vi "Channel Performance Test.vi"() -> ()   [LabVIEW 2021]
uses:
  CIFUtilities/CIFChannels/Typedef/Channel State.ctl
  <vilib>/Platform/TimedLoop/XDataNode/timing_clust.ctl
  <vilib>/Platform/TimedLoop/XDataNode/nitl_modes.ctl
  <vilib>/Platform/TimedLoop/XDataNode/wakeup.ctl
  Double/RTFIFODouble.lvclass/RTFIFODouble.ctl
  CIFUtilities/CIFChannels/CIFChannels.lvclass/CIFChannels.ctl
  ecd22e40-9ef3-47c9-84dd-6e51471c5b7d.vi
  cc845de9-9662-4d69-8494-93190ebbf16f.vi
  5dde9a10-7574-45f3-be33-437a2b751792.vi
  630e717b-411c-4f0a-96f3-098c02e0b307.vi
  27ef35cb-55c2-4e73-bad1-dda663d636b9.vi
  <vilib>/Utility/error.llb/Clear Errors.vi
  CIFUtilities/CIFChannels/Accessors/Write Channel State.vi
  CIFUtilities/CIFChannels/Accessors/Read Direction.vi
  ecd22e40-9ef3-47c9-84dd-6e51471c5b7d.vi/c28b0ead-42ad-4072-80a2-aca7f2bd7ce3.vi
  cc845de9-9662-4d69-8494-93190ebbf16f.vi/4bc1c15b-36ab-481f-b8dd-c64075ce723a.vi
  cc845de9-9662-4d69-8494-93190ebbf16f.vi/d83cb72b-7713-41fc-a3d1-682de79cf574.vi
  5dde9a10-7574-45f3-be33-437a2b751792.vi/c28b0ead-42ad-4072-80a2-aca7f2bd7ce3.vi
  630e717b-411c-4f0a-96f3-098c02e0b307.vi/c28b0ead-42ad-4072-80a2-aca7f2bd7ce3.vi
  630e717b-411c-4f0a-96f3-098c02e0b307.vi/219d0231-d98b-4193-b5cc-84f90e3c9091.vi
  27ef35cb-55c2-4e73-bad1-dda663d636b9.vi/c28b0ead-42ad-4072-80a2-aca7f2bd7ce3.vi
  27ef35cb-55c2-4e73-bad1-dda663d636b9.vi/219d0231-d98b-4193-b5cc-84f90e3c9091.vi
  Double/RTFIFODouble.lvclass
  D:/dev/CIF-LVCore/src/CIFUtilities/CIFChannels/CIFChannels.lvclass
  CIF-Core-LabVIEW/src/CIFServices/CIFServices Fill In Error Info Ex.vi
  <vilib>/Platform/TimedLoop/XDataNode/XDataNode.xnode
  <vilib>/Platform/TimedLoop/XDataNode/XDNodeRunTimeDep.lvlib
  CIF-Core-LabVIEW/src/CIFServices/CifChannelServices.lvlib
  CIFUtilities/CIFChannels/CIFChannels.lvclass
panel:
  out "avg RTFIFO 2":dbl
  out "Max RTFIFO 2":dbl
  out "Numeric 6":i32
  out "Numeric 5":dbl
  out "Numeric 4":dbl
  out "Channel State":T1
  out "Numeric 3":dbl
  out "Numeric 2":dbl
  out "Numeric":i32
  out "avg channel":dbl
  out "max channel":dbl
  out "avg RTFIFO":dbl
  out "Max RTFIFO":dbl
  out "pass":bool
  out "error out":errorcluster
  # "This test should be run on RT.  It stresses the communications by constantly creating resource contraints with the low priority sender and the high priority loop. On Windows the priority of the loops cannot be set."
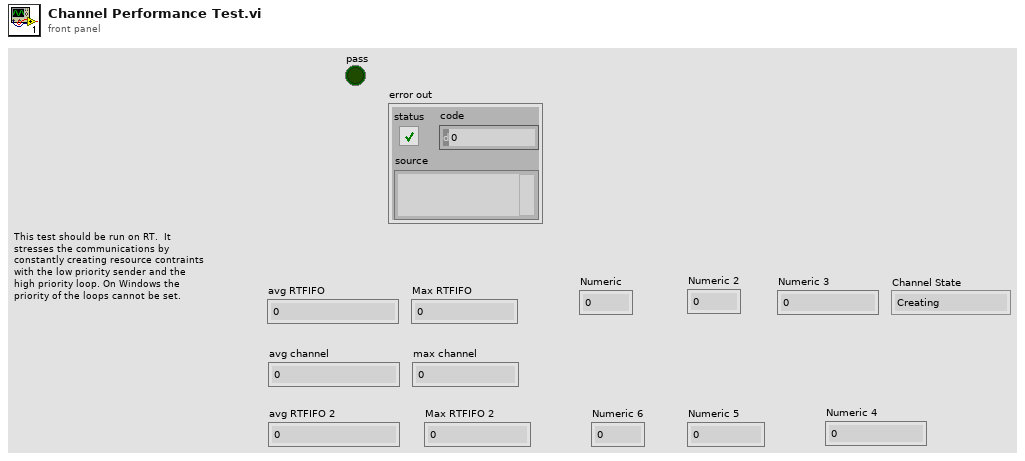
[diagram p1: front panel]
types:
  T1 = typedef "CIFChannels.lvclass/Channel State.ctl" = enum16{"Creating", "Disconnected", "Connecting", "Connected", "Destroying"}
  T2 = typedef "XDNodeRunTimeDep.lvlib/timing_clust.ctl" = cluster{"Expected End [f-1]":u64, "Actual End [f-1]":u64, "Finished Late? [f-1]":bool, "Expected End [i-1]":u64, "Actual End [i-1]":u64, "Finished Late? [i-1]":bool, "Expected Start [i]":u64, "Actual Start [i]":u64, "Expected Start [f]":u64, "Actual Start [f]":u64, "Source Name":string, "Structure Name":string, "Period":i64, "Deadline":i64, "Offset":i64, "Start":i64, "Priority":i32, "Timeout":i32, "Mode":T3, "Wakeup Reason":T4, "Error":errorcluster, "Source Type":string, "Secondary Source Type":string, "Global End Time":u64, "Global Start Time":u64, "Frame Duration":u64, "Iteration Duration":u64, "Assigned CPU":i32, "I/O Scan Engine Mode":u32}
  T3 = typedef "XDNodeRunTimeDep.lvlib/nitl_modes.ctl" = enum32{"No Change", "Process missed periods, maintain original phase", "Discard missed periods, maintain original phase", "Process missed periods, ignore original phase", "Discard missed periods, ignore original phase"}
  T4 = typedef "XDNodeRunTimeDep.lvlib/wakeup.ctl" = enum32{"Normal", "Aborted", "Asynchronous wakeup", "Timing source error", "Timed loop error", "Timeout"}
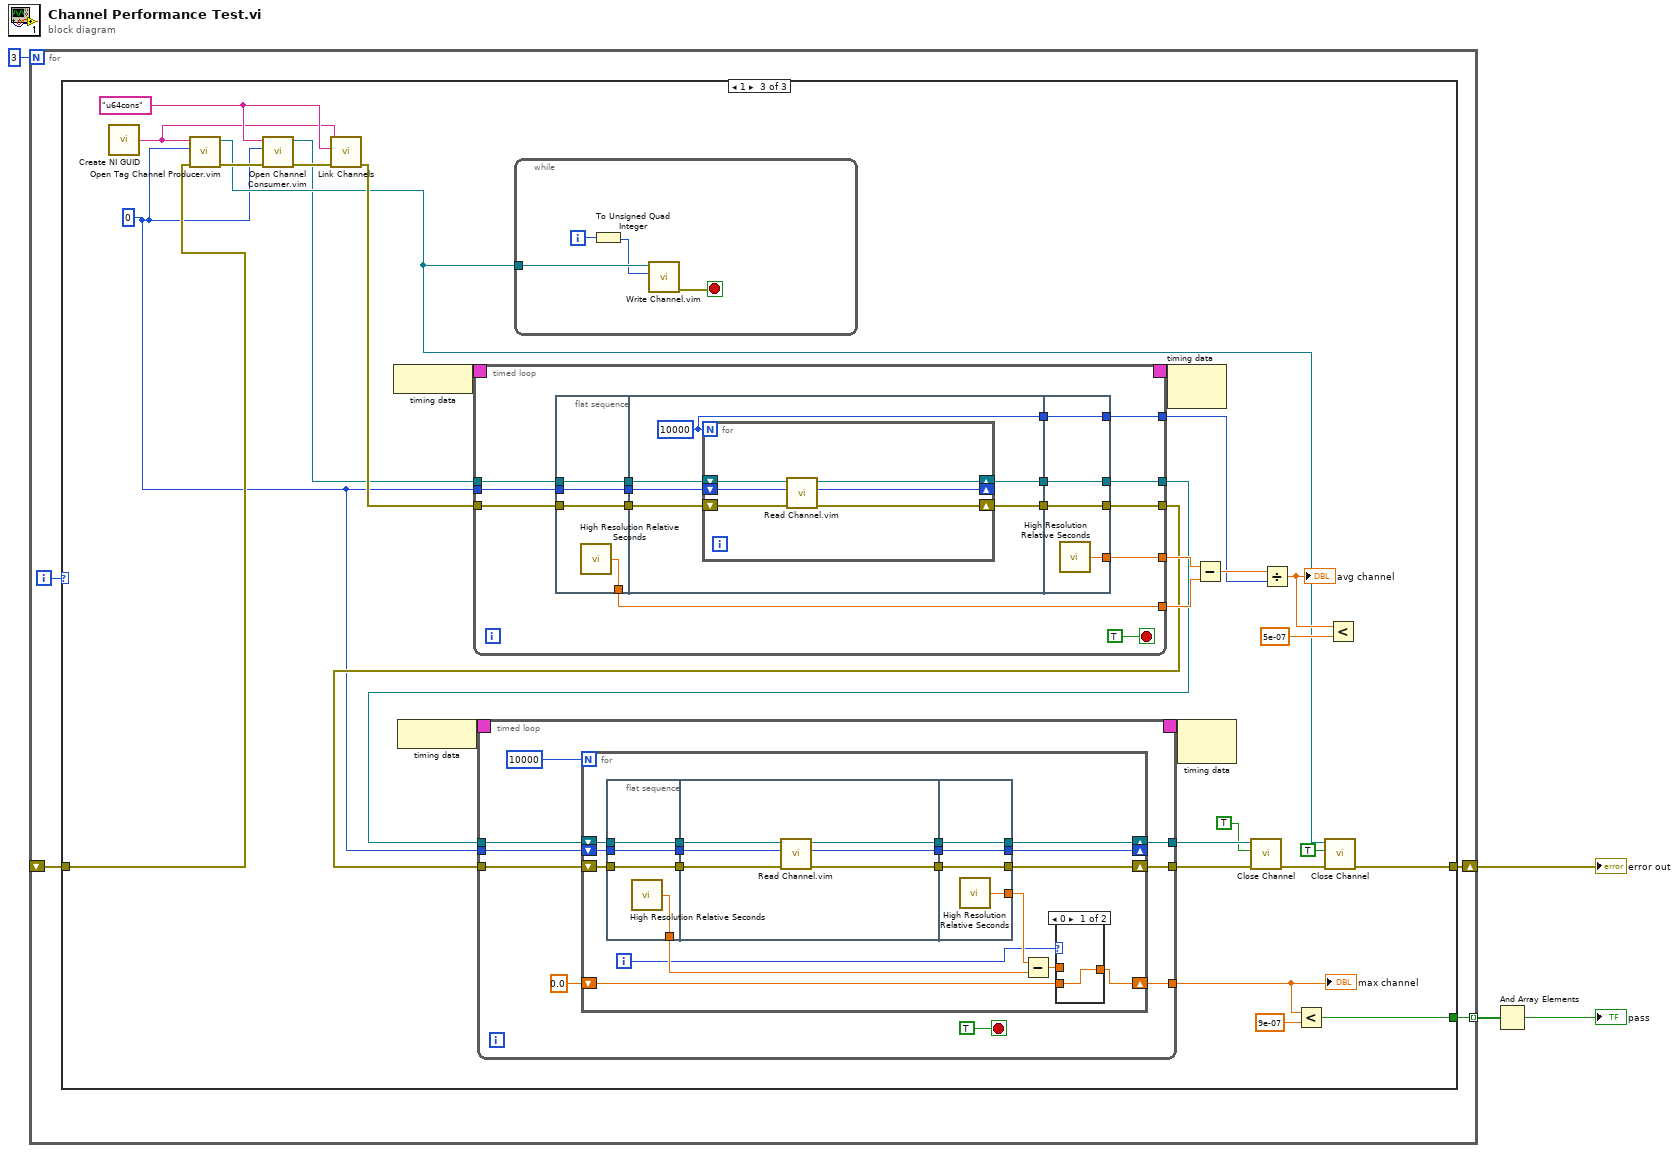
[diagram p0: block diagram]
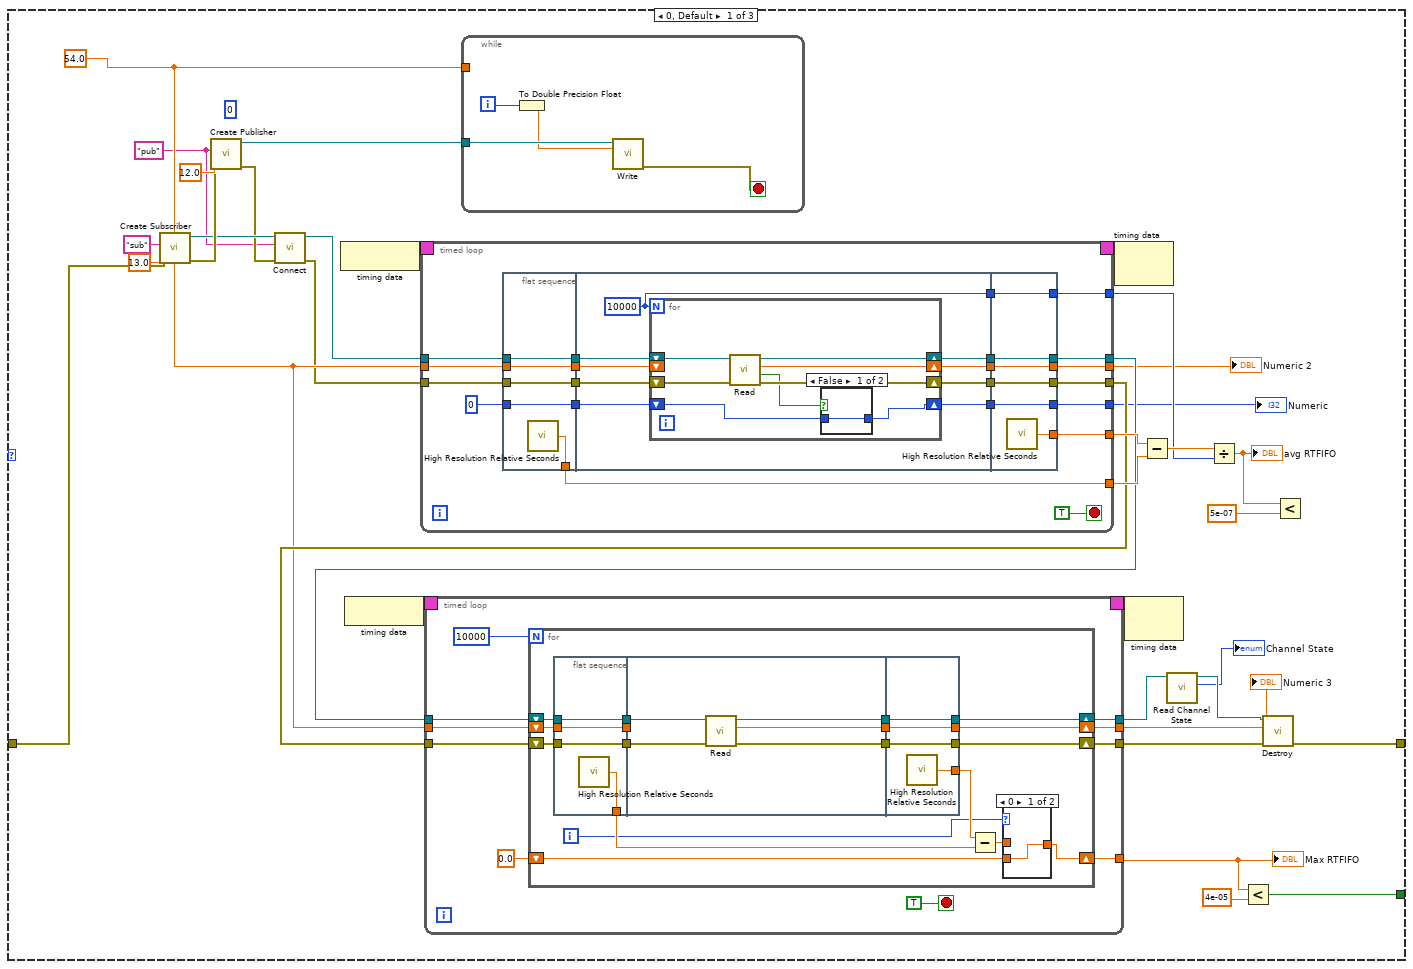
[diagram p2: hidden frame]
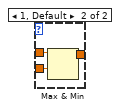
[diagram p3: hidden frame]
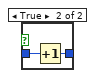
[diagram p4: hidden frame]
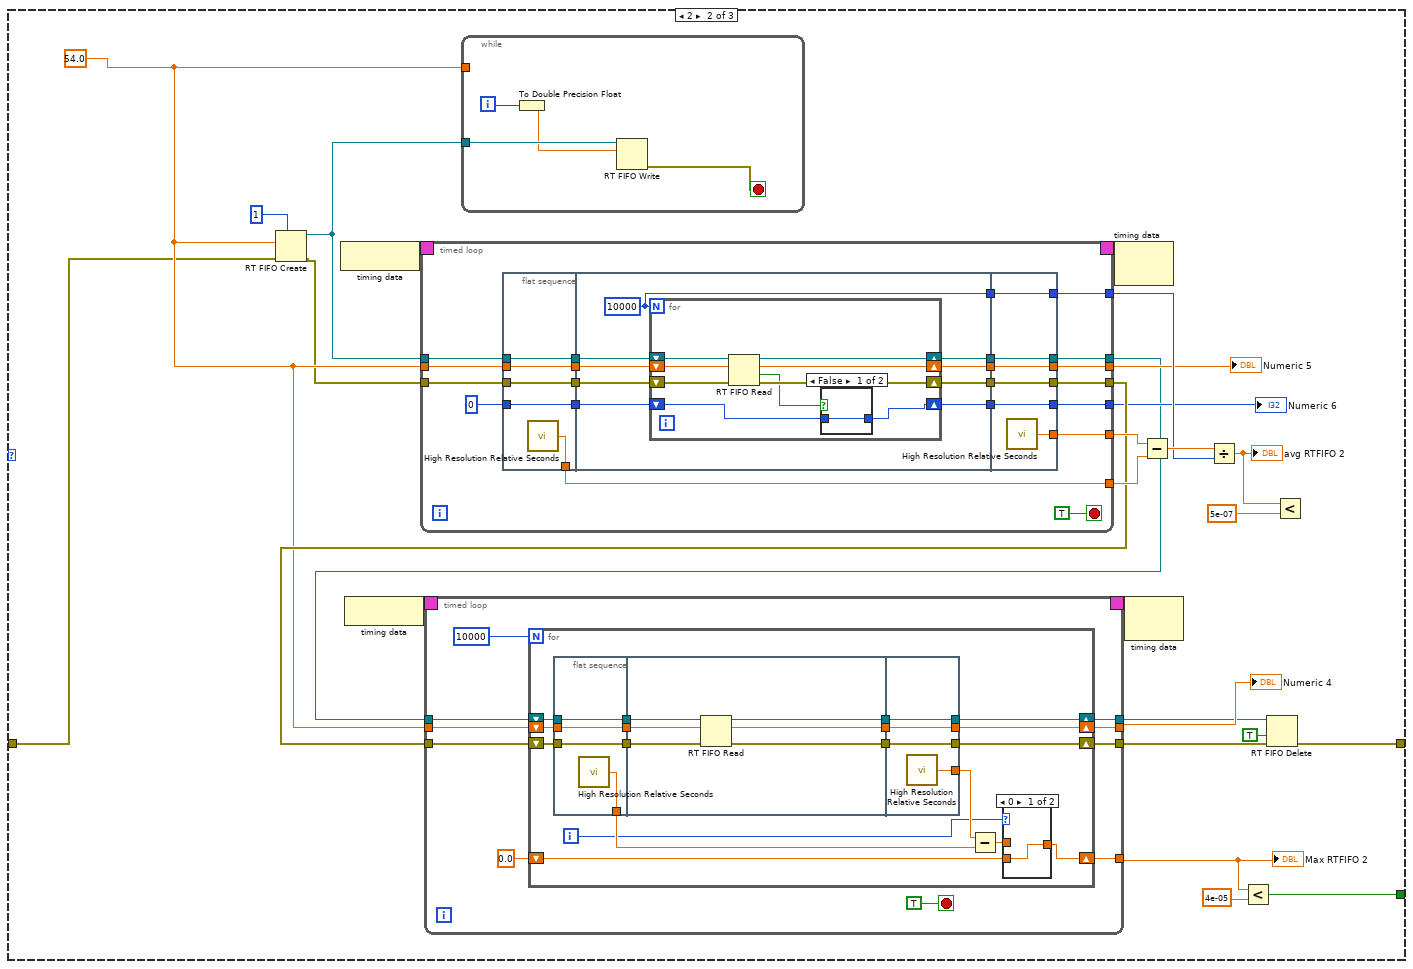
[diagram p5: hidden frame]
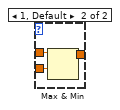
[diagram p6: hidden frame]
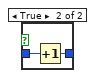
[diagram p7: hidden frame]
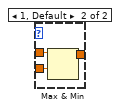
[diagram p8: hidden frame]
diagram:
  n1 = for {
    N: 3 -> [_]
    tunnel: [w8] -> w2 mode=indexing
    shift-right: [w7] -> w4
    shift-left: _ -> [w5]
    i -> [w6]
    n2 = case shown="1" w6 {
      tunnel: [w29 w166 w306] -> w8
      tunnel: [w15 w155 w296] -> w7
      tunnel: w5 -> [w22 w157 w301]
      frame 0, Default {
        w19 = "pub" ("Name")
        w28 = 54.0 ("Numeric")
        (unwired) u64 0
        n3 = call "Create Subscriber.vi"("error in (no error)"=w22, "Default Value"=13.0, "Name"="sub") -> ("error out"=w23:errorcluster, "RTFIFODouble out"=w21:refnum<class "RTFIFODouble.lvclass">)  [unwired: 7 in]
        n4 = call "Create Publisher.vi"("error in (no error)"=w23, "Default Value"=12.0, "Name"=w19) -> ("error out"=w20:errorcluster, "RTFIFODouble out"=w24:refnum<class "RTFIFODouble.lvclass">)  [unwired: 7 in]
        n5 = call-dynamic "Connect.vi"("error in (no error)"=w20, "Connection Name"=w19, "RTFIFODouble in"=w21) -> ("error out"=w17:errorcluster, "RTFIFODouble out"=w18:refnum<class "RTFIFODouble.lvclass">)  [unwired: 7 in]
        n6 = node-c288() -> (w43:T2)
        n7 = node-c288() -> (w41:T2)
        n8 = timed-loop {
          timing: w43 -> [_]
          timing-out: [_] -> w42
          tunnel: w18 -> [w117]
          tunnel: w17 -> [w116]
          tunnel: [w112] -> w35
          tunnel: [w110] -> w34
          tunnel: [w108] -> w39
          tunnel: [w107] -> w38
          tunnel: [w106] -> w36
          tunnel: w28 -> [w104]
          tunnel: [w100] -> w14
          tunnel: [w98] -> w13
          stop <- TRUE stop-if-true
          n9 = flat-sequence {
            tunnel: w116 -> [w121]
            tunnel: w117 -> [w122]
            tunnel: [w122] -> w114
            tunnel: [w121] -> w113
            tunnel: [w120] -> w107
            tunnel: w104 -> [w119]
            tunnel: [w119] -> w103
            tunnel: [w118] -> w102
            tunnel: 0 -> [w118]
            tunnel: w114 -> [w131]
            tunnel: w113 -> [w130]
            tunnel: [w129] -> w111
            tunnel: [w128] -> w109
            tunnel: [w127] -> w105
            tunnel: w103 -> [w126]
            tunnel: w102 -> [w125]
            tunnel: [w124] -> w99
            tunnel: [w123] -> w97
            tunnel: [w148] -> w112
            tunnel: w111 -> [w148]
            tunnel: [w147] -> w110
            tunnel: w109 -> [w147]
            tunnel: [w146] -> w108
            tunnel: [w145] -> w106
            tunnel: w105 -> [w145]
            tunnel: [w144] -> w100
            tunnel: w99 -> [w144]
            tunnel: [w143] -> w98
            tunnel: w97 -> [w143]
            frame #0 {
              n10 = call <vilib>:"High Resolution Relative Seconds.vi"() -> ("relative seconds"=w120:dbl)
            }
            frame #1 {
              w127 = 10000
              n11 = for {
                N: w127 -> [_]
                shift-right: [w137] -> w129
                shift-left: w131 -> [w139]
                shift-right: [w136] -> w128
                shift-left: w130 -> [w138]
                shift-right: [w135] -> w123
                shift-left: w126 -> [_]
                shift-right: [w132] -> w124
                shift-left: w125 -> [w133]
                n12 = call "Read.vi"("error in (no error)"=w138, "RTFIFODouble in"=w139) -> ("error out"=w136:errorcluster, "timed out?"=w134:bool, "Data"=w135:dbl, "RTFIFODouble out"=w137:refnum<class "RTFIFODouble.lvclass">)  [unwired: 6 in]
                n13 = case shown="False" w134 {
                  tunnel: w133 -> [w140 w142]
                  tunnel: [w140 w141] -> w132
                  frame False {
                  }
                  frame True {
                    n14 = Increment(x=w142) -> (x+1=w141:i32)
                  }
                }
              }
            }
            frame #2 {
              n15 = call <vilib>:"High Resolution Relative Seconds.vi"() -> ("relative seconds"=w146:dbl)
            }
          }
        }
        "Numeric" <- w14
        "Numeric 2" <- w13
        n16 = timed-loop {
          timing: w41 -> [_]
          timing-out: [_] -> w40
          tunnel: w35 -> [w57]
          tunnel: w34 -> [w56]
          tunnel: [w54] -> w11
          tunnel: [w53] -> w16
          tunnel: w28 -> [w52]
          tunnel: [w49] -> w31
          tunnel: [w48] -> w12
          stop <- TRUE stop-if-true
          n17 = for {
            N: 10000 -> [_]
            shift-right: [w69] -> w54
            shift-left: w57 -> [w71]
            shift-right: [w68] -> w53
            shift-left: w56 -> [w70]
            shift-right: [w62] -> w49
            shift-left: 0.0 -> [w63]
            shift-right: [w61] -> w48
            shift-left: w52 -> [w67]
            i -> [w59]
            n18 = flat-sequence {
              tunnel: w70 -> [w82]
              tunnel: w71 -> [w83]
              tunnel: [w83] -> w75
              tunnel: [w82] -> w74
              tunnel: [w81] -> w65
              tunnel: w67 -> [w80]
              tunnel: [w80] -> w73
              tunnel: w75 -> [w88]
              tunnel: w74 -> [w87]
              tunnel: [w86] -> w72
              tunnel: w73 -> [_]
              tunnel: [w84] -> w60
              tunnel: [w85] -> w58
              tunnel: [w92] -> w69
              tunnel: w72 -> [w92]
              tunnel: [w91] -> w68
              tunnel: [w90] -> w66
              tunnel: [w89] -> w61
              tunnel: w60 -> [w89]
              tunnel: w58 -> [w91]
              frame #0 {
                n19 = call <vilib>:"High Resolution Relative Seconds.vi"() -> ("relative seconds"=w81:dbl)
              }
              frame #1 {
                n20 = call "Read.vi"("error in (no error)"=w87, "RTFIFODouble in"=w88) -> ("error out"=w85:errorcluster, "Data"=w84:dbl, "RTFIFODouble out"=w86:refnum<class "RTFIFODouble.lvclass">)  [unwired: 6 in, 1 out]
              }
              frame #2 {
                n21 = call <vilib>:"High Resolution Relative Seconds.vi"() -> ("relative seconds"=w90:dbl)
              }
            }
            n22 = Subtract(x=w66, y=w65) -> (x-y=w64:dbl)
            n23 = case shown="0" w59 {
              tunnel: w64 -> [_ w79]
              tunnel: w63 -> [w76 w78]
              tunnel: [w76 w77] -> w62
              frame 0 {
              }
              frame 1, Default {
                n24 = Max & Min(x=w79, y=w78) -> (max(x,y)=w77:dbl)  [unwired: 1 out]
              }
            }
          }
        }
        "Max RTFIFO" <- w31
        "Numeric 3" <- w12
        n25 = while {
          tunnel: w24 -> [w47]
          tunnel: w28 -> [_]
          i -> [w45]
          stop <- w46 stop-if-true
          n26 = To Double Precision Float(number=w45) -> (double precision float=w44:dbl)
          n27 = call "Write.vi"("Data"=w44, "RTFIFODouble in"=w47) -> ("error out"=w46:errorcluster)  [unwired: 7 in, 2 out]
        }
        n28 = node-c288(w42) -> ()  [unwired: 1 out]
        n29 = node-c288(w40) -> ()  [unwired: 1 out]
        n30 = Subtract(x=w39, y=w38) -> (x-y=w37:dbl)
        n31 = call "Read Channel State.vi"("CIFChannels in"=w11) -> ("Channel State"=→"Channel State":T1, "CIFChannels out"=w10:refnum<class "RTFIFODouble.lvclass">)  [unwired: 8 in, 1 out]
        n32 = Divide(x=w37, y=w36) -> (x/y=w33:dbl)
        "avg RTFIFO" <- w33
        n33 = Less?(x=w31, y=4e-05) -> (x < y?=w29:bool)
        n34 = call-dynamic "Destroy.vi"("error in (no error)"=w16, "RTFIFODouble in"=w10) -> ("error out"=w15:errorcluster)  [unwired: 8 in, 1 out]
        n35 = Less?(x=w33, y=5e-07) -> ()  [unwired: 1 out]
      }
      frame 2 {
        w163 = 54.0 ("Numeric")
        n36 = RT FIFO Create(1:w163, 3:w157, 4:u32 1 ("size (10)")) -> (8:w158:refnum<k33>, 11:w159:errorcluster)  [unwired: 5 in, 1 out]
        n37 = node-c288() -> (w179:T2)
        n38 = node-c288() -> (w177:T2)
        n39 = timed-loop {
          timing: w179 -> [_]
          timing-out: [_] -> w178
          tunnel: w158 -> [w254]
          tunnel: w159 -> [w253]
          tunnel: [w249] -> w160
          tunnel: [w247] -> w171
          tunnel: [w245] -> w175
          tunnel: [w244] -> w174
          tunnel: [w243] -> w172
          tunnel: w163 -> [w241]
          tunnel: [w237] -> w165
          tunnel: [w235] -> w164
          stop <- TRUE stop-if-true
          n40 = flat-sequence {
            tunnel: w253 -> [w258]
            tunnel: w254 -> [w259]
            tunnel: [w259] -> w251
            tunnel: [w258] -> w250
            tunnel: [w257] -> w244
            tunnel: w241 -> [w256]
            tunnel: [w256] -> w240
            tunnel: [w255] -> w239
            tunnel: 0 -> [w255]
            tunnel: w251 -> [w268]
            tunnel: w250 -> [w267]
            tunnel: [w266] -> w248
            tunnel: [w265] -> w246
            tunnel: [w264] -> w242
            tunnel: w240 -> [w263]
            tunnel: w239 -> [w262]
            tunnel: [w261] -> w236
            tunnel: [w260] -> w234
            tunnel: [w286] -> w249
            tunnel: w248 -> [w286]
            tunnel: [w285] -> w247
            tunnel: w246 -> [w285]
            tunnel: [w284] -> w245
            tunnel: [w283] -> w243
            tunnel: w242 -> [w283]
            tunnel: [w282] -> w237
            tunnel: w236 -> [w282]
            tunnel: [w281] -> w235
            tunnel: w234 -> [w281]
            frame #0 {
              n41 = call <vilib>:"High Resolution Relative Seconds.vi"() -> ("relative seconds"=w257:dbl)
            }
            frame #1 {
              w264 = 10000
              n42 = for {
                N: w264 -> [_]
                shift-right: [w274] -> w266
                shift-left: w268 -> [w275]
                shift-right: [w271] -> w265
                shift-left: w267 -> [w272]
                shift-right: [w270] -> w260
                shift-left: w263 -> [w273]
                shift-right: [w276] -> w261
                shift-left: w262 -> [w277]
                n43 = RT FIFO Read(0:w275, 1:w273, 3:w272) -> (8:w274:refnum<k33>, 9:w270:dbl, 10:w269:bool, 11:w271:errorcluster)  [unwired: 1 in, 1 out]
                n44 = case shown="False" w269 {
                  tunnel: w277 -> [w278 w280]
                  tunnel: [w278 w279] -> w276
                  frame False {
                  }
                  frame True {
                    n45 = Increment(x=w280) -> (x+1=w279:i32)
                  }
                }
              }
            }
            frame #2 {
              n46 = call <vilib>:"High Resolution Relative Seconds.vi"() -> ("relative seconds"=w284:dbl)
            }
          }
        }
        "Numeric 6" <- w165
        "Numeric 5" <- w164
        n47 = timed-loop {
          timing: w177 -> [_]
          timing-out: [_] -> w176
          tunnel: w160 -> [w193]
          tunnel: w171 -> [w192]
          tunnel: [w190] -> w156
          tunnel: w163 -> [w189]
          tunnel: [w186] -> w168
          tunnel: [w185] -> w161
          tunnel: [w184] -> w154
          stop <- TRUE stop-if-true
          n48 = for {
            N: 10000 -> [_]
            shift-right: [w205] -> w184
            shift-left: w193 -> [w207]
            shift-right: [w204] -> w190
            shift-left: w192 -> [w206]
            shift-right: [w198] -> w186
            shift-left: 0.0 -> [w199]
            shift-right: [w197] -> w185
            shift-left: w189 -> [w203]
            i -> [w195]
            n49 = flat-sequence {
              tunnel: w206 -> [w218]
              tunnel: w207 -> [w219]
              tunnel: [w219] -> w211
              tunnel: [w218] -> w210
              tunnel: [w217] -> w201
              tunnel: w203 -> [w216]
              tunnel: [w216] -> w209
              tunnel: w211 -> [w221]
              tunnel: w210 -> [w224]
              tunnel: [w222] -> w208
              tunnel: w209 -> [w225]
              tunnel: [w220] -> w196
              tunnel: [w223] -> w194
              tunnel: [w229] -> w205
              tunnel: w208 -> [w229]
              tunnel: [w228] -> w204
              tunnel: [w227] -> w202
              tunnel: [w226] -> w197
              tunnel: w196 -> [w226]
              tunnel: w194 -> [w228]
              frame #0 {
                n50 = call <vilib>:"High Resolution Relative Seconds.vi"() -> ("relative seconds"=w217:dbl)
              }
              frame #1 {
                n51 = RT FIFO Read(0:w221, 1:w225, 3:w224) -> (8:w222:refnum<k33>, 9:w220:dbl, 11:w223:errorcluster)  [unwired: 1 in, 2 out]
              }
              frame #2 {
                n52 = call <vilib>:"High Resolution Relative Seconds.vi"() -> ("relative seconds"=w227:dbl)
              }
            }
            n53 = Subtract(x=w202, y=w201) -> (x-y=w200:dbl)
            n54 = case shown="0" w195 {
              tunnel: w200 -> [_ w215]
              tunnel: w199 -> [w212 w214]
              tunnel: [w212 w213] -> w198
              frame 0 {
              }
              frame 1, Default {
                n55 = Max & Min(x=w215, y=w214) -> (max(x,y)=w213:dbl)  [unwired: 1 out]
              }
            }
          }
        }
        "Max RTFIFO 2" <- w168
        "Numeric 4" <- w161
        n56 = while {
          tunnel: w158 -> [w182]
          tunnel: w163 -> [_]
          i -> [w183]
          stop <- w180 stop-if-true
          n57 = To Double Precision Float(number=w183) -> (double precision float=w181:dbl)
          n58 = RT FIFO Write(0:w182, 1:w181) -> (11:w180:errorcluster)  [unwired: 3 in, 3 out]
        }
        n59 = node-c288(w178) -> ()  [unwired: 1 out]
        n60 = node-c288(w176) -> ()  [unwired: 1 out]
        n61 = Subtract(x=w175, y=w174) -> (x-y=w173:dbl)
        n62 = Divide(x=w173, y=w172) -> (x/y=w170:dbl)
        "avg RTFIFO 2" <- w170
        n63 = Less?(x=w168, y=4e-05) -> (x < y?=w166:bool)
        n64 = RT FIFO Delete(0:w154, 2:TRUE ("force destroy? (F)"), 3:w156) -> (11:w155:errorcluster)
        n65 = Less?(x=w170, y=5e-07) -> ()  [unwired: 1 out]
      }
      frame 1 {
        w303 = "u64cons" ("Channel Name")
        w291 = u64 0
        n66 = call <vilib>:"Create NI GUID.vi"() -> ("NI GUID"=w294:string)
        n67 = call "Open Tag Channel Producer.vim"("error in"=w301, "Input Type"=w291, "Channel Name"=w294) -> ("error out"=w305:errorcluster, "ADAS HIL Channel"=w295:refnum<k21>)  [unwired: 7 in]
        n68 = call "Open Channel Consumer.vim"("error in"=w305, "Input Type"=w291, "Channel Name"=w303) -> ("error out"=w304:errorcluster, "ADAS HIL Channel"=w292:refnum<k21>)  [unwired: 7 in]
        n69 = call "Link Channels.vi"("error in"=w304, "Consumer Channel Name"=w303, "Producer Channel Name"=w294) -> ("error out"=w302:errorcluster)  [unwired: 8 in]
        n70 = node-c288() -> (w320:T2)
        n71 = node-c288() -> (w318:T2)
        n72 = timed-loop {
          timing: w320 -> [_]
          timing-out: [_] -> w319
          tunnel: w292 -> [w388]
          tunnel: w302 -> [w387]
          tunnel: [w383] -> w312
          tunnel: [w381] -> w311
          tunnel: [w379] -> w316
          tunnel: [w378] -> w315
          tunnel: [w377] -> w313
          tunnel: w291 -> [w375]
          stop <- TRUE stop-if-true
          n73 = flat-sequence {
            tunnel: w387 -> [w391]
            tunnel: w388 -> [w392]
            tunnel: [w392] -> w385
            tunnel: [w391] -> w384
            tunnel: [w390] -> w378
            tunnel: w375 -> [w389]
            tunnel: [w389] -> w374
            tunnel: w385 -> [w398]
            tunnel: w384 -> [w397]
            tunnel: [w396] -> w382
            tunnel: [w395] -> w380
            tunnel: [w394] -> w376
            tunnel: w374 -> [w393]
            tunnel: [w408] -> w383
            tunnel: w382 -> [w408]
            tunnel: [w407] -> w381
            tunnel: w380 -> [w407]
            tunnel: [w406] -> w379
            tunnel: [w405] -> w377
            tunnel: w376 -> [w405]
            frame #0 {
              n74 = call <vilib>:"High Resolution Relative Seconds.vi"() -> ("relative seconds"=w390:dbl)
            }
            frame #1 {
              w394 = 10000
              n75 = for {
                N: w394 -> [_]
                shift-right: [w401] -> w396
                shift-left: w398 -> [w404]
                shift-right: [w400] -> w395
                shift-left: w397 -> [w399]
                shift-right: [w402] -> _
                shift-left: w393 -> [w403]
                n76 = call "Read Channel.vim"("error in"=w399, "Data in"=w403, "ADAS HIL Channel in"=w404) -> ("error out"=w400:errorcluster, "Data out"=w402:u64, "ADAS HIL Channel out"=w401:refnum<k21>)  [unwired: 5 in, 1 out]
              }
            }
            frame #2 {
              n77 = call <vilib>:"High Resolution Relative Seconds.vi"() -> ("relative seconds"=w406:dbl)
            }
          }
        }
        n78 = timed-loop {
          timing: w318 -> [_]
          timing-out: [_] -> w317
          tunnel: w312 -> [w333]
          tunnel: w311 -> [w332]
          tunnel: [w330] -> w299
          tunnel: [w329] -> w300
          tunnel: w291 -> [w328]
          tunnel: [w325] -> w308
          stop <- TRUE stop-if-true
          n79 = for {
            N: 10000 -> [_]
            shift-right: [w345] -> w330
            shift-left: w333 -> [w347]
            shift-right: [w344] -> w329
            shift-left: w332 -> [w346]
            shift-right: [w338] -> w325
            shift-left: 0.0 -> [w339]
            shift-right: [w337] -> _
            shift-left: w328 -> [w343]
            i -> [w335]
            n80 = flat-sequence {
              tunnel: w346 -> [w358]
              tunnel: w347 -> [w359]
              tunnel: [w359] -> w351
              tunnel: [w358] -> w350
              tunnel: [w357] -> w341
              tunnel: w343 -> [w356]
              tunnel: [w356] -> w349
              tunnel: w351 -> [w365]
              tunnel: w350 -> [w361]
              tunnel: [w364] -> w348
              tunnel: w349 -> [w363]
              tunnel: [w362] -> w336
              tunnel: [w360] -> w334
              tunnel: [w369] -> w345
              tunnel: w348 -> [w369]
              tunnel: [w368] -> w344
              tunnel: [w367] -> w342
              tunnel: [w366] -> w337
              tunnel: w336 -> [w366]
              tunnel: w334 -> [w368]
              frame #0 {
                n81 = call <vilib>:"High Resolution Relative Seconds.vi"() -> ("relative seconds"=w357:dbl)
              }
              frame #1 {
                n82 = call "Read Channel.vim"("error in"=w361, "Data in"=w363, "ADAS HIL Channel in"=w365) -> ("error out"=w360:errorcluster, "Data out"=w362:u64, "ADAS HIL Channel out"=w364:refnum<k21>)  [unwired: 5 in, 1 out]
              }
              frame #2 {
                n83 = call <vilib>:"High Resolution Relative Seconds.vi"() -> ("relative seconds"=w367:dbl)
              }
            }
            n84 = Subtract(x=w342, y=w341) -> (x-y=w340:dbl)
            n85 = case shown="0" w335 {
              tunnel: w340 -> [_ w355]
              tunnel: w339 -> [w352 w354]
              tunnel: [w352 w353] -> w338
              frame 0 {
              }
              frame 1, Default {
                n86 = Max & Min(x=w355, y=w354) -> (max(x,y)=w353:dbl)  [unwired: 1 out]
              }
            }
          }
        }
        "max channel" <- w308
        n87 = while {
          tunnel: w295 -> [w323]
          i -> [w324]
          stop <- w321 stop-if-true
          n88 = To Unsigned Quad Integer(1:w324) -> (0:w322:u64)
          n89 = call "Write Channel.vim"("Data in"=w322, "ADAS HIL Channel in"=w323) -> ("error out"=w321:errorcluster)  [unwired: 7 in, 2 out]
        }
        n90 = node-c288(w319) -> ()  [unwired: 1 out]
        n91 = node-c288(w317) -> ()  [unwired: 1 out]
        n92 = Subtract(x=w316, y=w315) -> (x-y=w314:dbl)
        n93 = call "Close Channel.vi"("error in"=w300, "Force Destroy? (F)"=TRUE, "ADAS HIL Channel"=w299) -> ("error out"=w298:errorcluster)  [unwired: 8 in]
        n94 = Divide(x=w314, y=w313) -> (x/y=w310:dbl)
        "avg channel" <- w310
        n95 = Less?(x=w308, y=9e-07) -> (x < y?=w306:bool)
        n96 = call "Close Channel.vi"("error in"=w298, "Force Destroy? (F)"=TRUE, "ADAS HIL Channel"=w295) -> ("error out"=w296:errorcluster)  [unwired: 8 in]
        n97 = Less?(x=w310, y=5e-07) -> ()  [unwired: 1 out]
      }
    }
  }
  "error out" <- w4
  n98 = And Array Elements(Boolean array=w2) -> (logical AND=→"pass":bool)
